vi "Example_chartsheet.vi"() -> ()   [LabVIEW 8.6]
uses:
  Controls/lxw_chart_marker_type.ctl
  Controls/lxw_chart_legend_position.ctl
  Controls/lxw_chart_axis_type.ctl
  Controls/lxw_chart_type.ctl
panel:
  out "function return 2":string
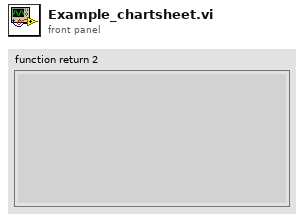
[diagram p1: front panel]
types:
  T1 = enum32{"invalid app kind", "Development System", "Run Time System", "Student Edition", "Embedded LabVIEW", "Evaluation", "Custom"}
  T2 = cluster{"color":u32, "none":u8, "@dummy control@":i8, "@dummy control@":i8, "@dummy control@":i8, "width":sgl, "dash_type":u8, "transparency":u8}
  T3 = cluster{"color":u32, "none":u8, "transparency":u8}
  T4 = typedef "lxw_chart_type.ctl" = u8
  T5 = typedef "lxw_chart_axis_type.ctl" = u8
  T6 = typedef "lxw_chart_legend_position.ctl" = u8
  T7 = typedef "lxw_chart_marker_type.ctl" = u8
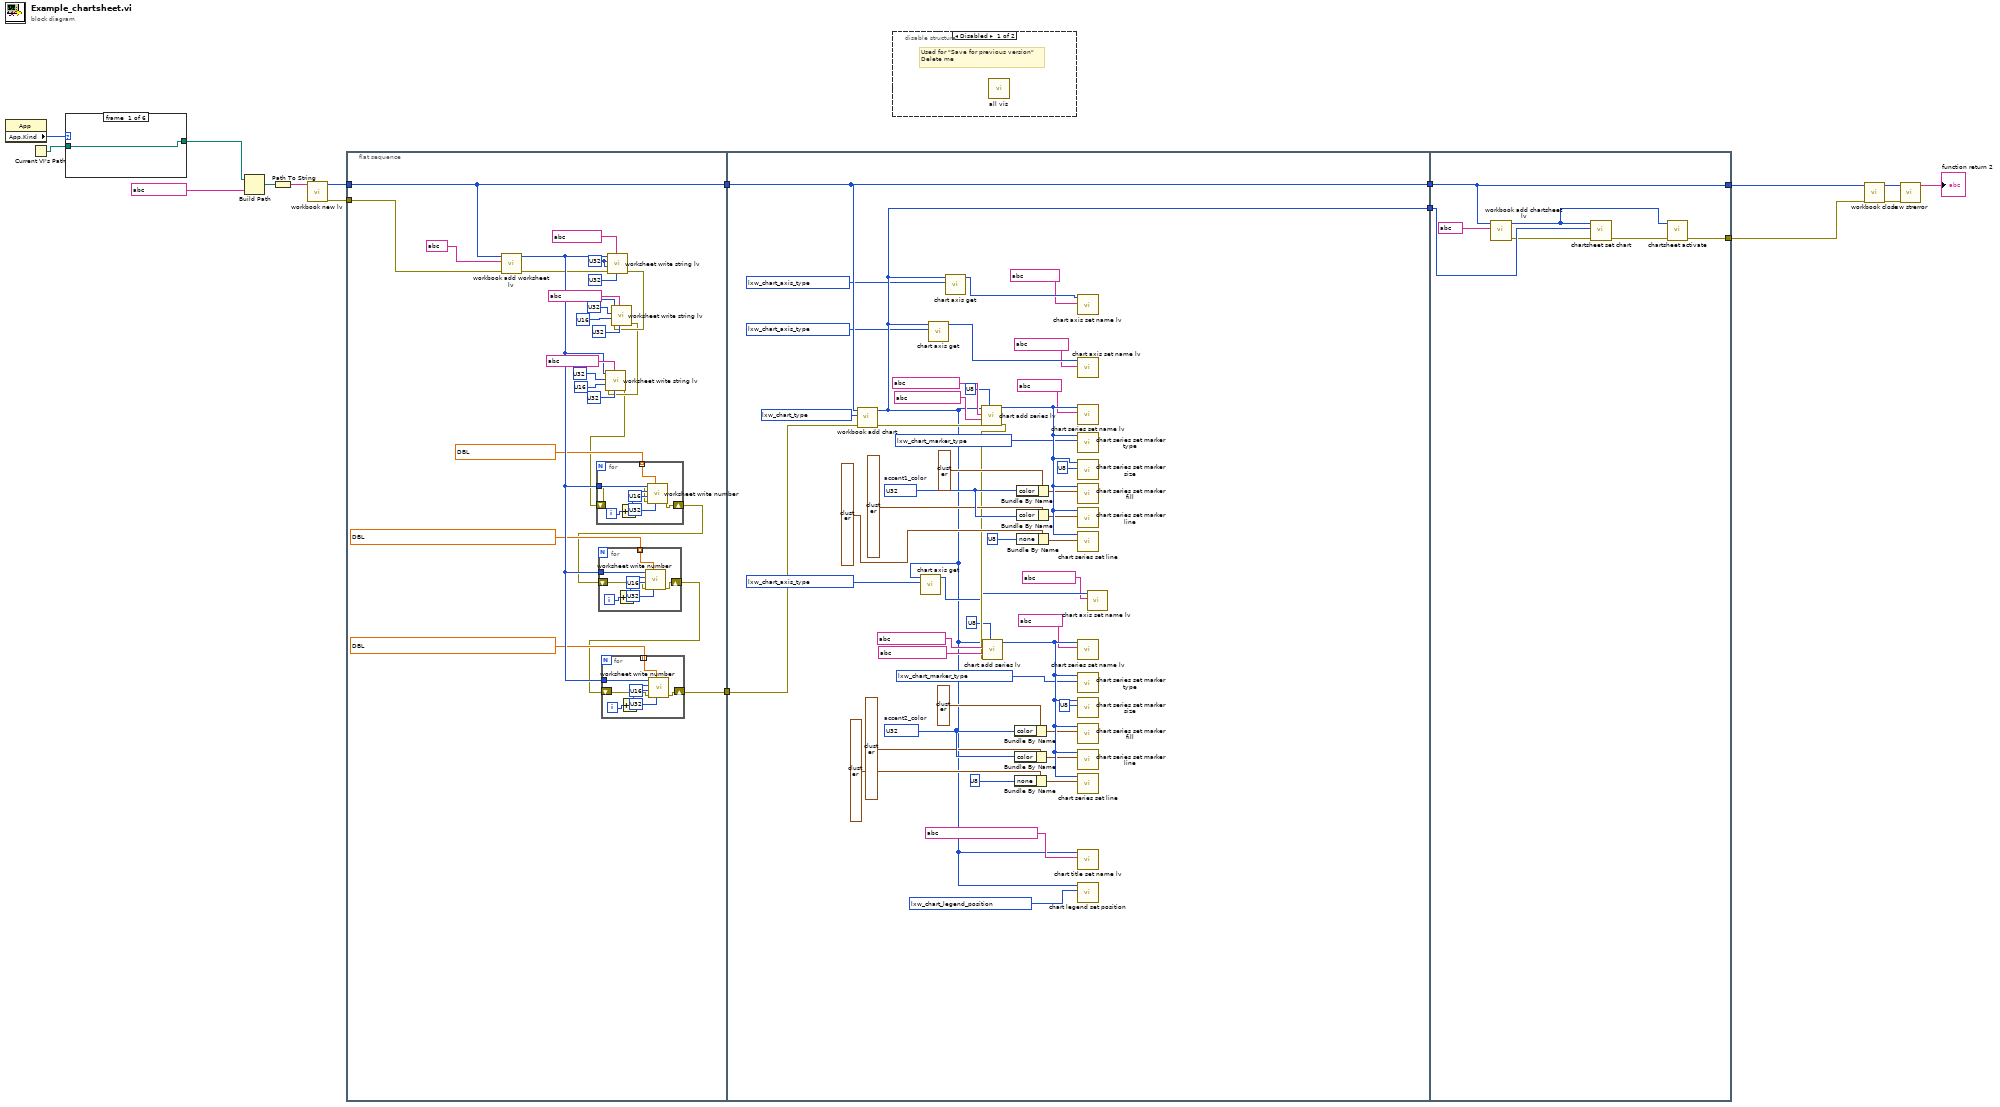
[diagram p0: block diagram]
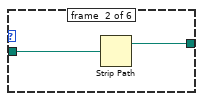
[diagram p2: hidden frame]
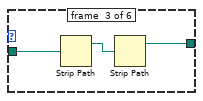
[diagram p3: hidden frame]
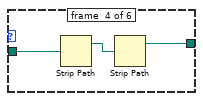
[diagram p4: hidden frame]
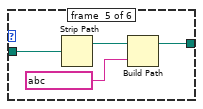
[diagram p5: hidden frame]
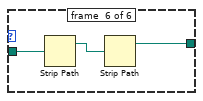
[diagram p6: hidden frame]
diagram:
  n1 = property class="App"() -> ("App.Kind"=w6:T1)  [unwired: 2 in, 2 out]
  n2 = Current VI's Path() -> (path=w5:path)
  n3 = case shown="\"Evaluation\"" w6 {
    tunnel: w5 -> [w18 w20 w23 w26 w30 w33]
    tunnel: [w18 w19 w21 w24 w28 w31] -> w3
    frame #0 {
    }
    frame #1 {
      n4 = Strip Path(path=w20) -> (stripped path=w19:path)  [unwired: 1 out]
    }
    frame #2 {
      n5 = Strip Path(path=w23) -> (stripped path=w22:path)  [unwired: 1 out]
      n6 = Strip Path(path=w22) -> (stripped path=w21:path)  [unwired: 1 out]
    }
    frame #3 {
      n7 = Strip Path(path=w26) -> (stripped path=w25:path)  [unwired: 1 out]
      n8 = Strip Path(path=w25) -> (stripped path=w24:path)  [unwired: 1 out]
    }
    frame #4 {
      n9 = Strip Path(path=w30) -> (stripped path=w29:path)  [unwired: 1 out]
      n10 = Build Path(base path=w29, name or relative path=string ?) -> (appended path=w28:path)
    }
    frame #5 {
      n11 = Strip Path(path=w33) -> (stripped path=w32:path)  [unwired: 1 out]
      n12 = Strip Path(path=w32) -> (stripped path=w31:path)  [unwired: 1 out]
    }
  }
  n13 = Build Path(base path=w3, name or relative path=string ? ("filename")) -> (appended path=w2:path)
  n14 = Path To String(path=w2) -> (string=w1:string)
  n15 = call "workbook new lv.vi"("filename"=w1) -> ("error out"=w14:errorcluster, "function return"=w17:u32)  [unwired: 9 in]
  n16 = flat-sequence {
    tunnel: w17 -> [w36]
    tunnel: w14 -> [w35]
    tunnel: [w37] -> w13
    tunnel: [w36] -> w12
    tunnel: w13 -> [w108]
    tunnel: w12 -> [w109]
    tunnel: [w109] -> w10
    tunnel: [w88] -> w9
    tunnel: [w135] -> w11
    tunnel: w10 -> [w133]
    tunnel: w9 -> [w134]
    tunnel: [w133] -> w8
    frame #0 {
      w57 = u32 ? ("row")
      n17 = call "workbook add worksheet lv.vi"("error in (no error)"=w35, "sheetname"=string ?, "workbook"=w36) -> ("error out"=w34:errorcluster, "function return"=w46:u32)  [unwired: 7 in]
      n18 = call "worksheet write string lv.vi"("format"=u32 ?, "string"=string ?, "error in (no error)"=w34, "col"=w57, "row"=w57, "worksheet"=w46) -> ("error out"=w42:errorcluster)  [unwired: 4 in, 1 out]
      n19 = call "worksheet write string lv.vi"("format"=u32 ?, "string"=string ?, "error in (no error)"=w42, "col"=u16 ?, "row"=u32 ?, "worksheet"=w46) -> ("error out"=w41:errorcluster)  [unwired: 4 in, 1 out]
      n20 = call "worksheet write string lv.vi"("format"=u32 ?, "string"=string ?, "error in (no error)"=w41, "col"=u16 ?, "row"=u32 ?, "worksheet"=w46) -> ("error out"=w40:errorcluster)  [unwired: 4 in, 1 out]
      n21 = for {
        tunnel: w46 -> [w82]
        tunnel: dbl[] ? -> [w81] mode=indexing
        shift-right: [w75] -> w39
        shift-left: w40 -> [w76]
        i -> [w80]
        n22 = Increment(x=w80) -> (x+1=w79:i32)
        n23 = call "worksheet write number.vi"("format"=u32 ?, "number"=w81, "error in (no error)"=w76, "col"=u16 ?, "row"=w79, "worksheet"=w82) -> ("error out"=w75:errorcluster)  [unwired: 4 in, 1 out]
      }
      n24 = for {
        tunnel: w46 -> [w74]
        tunnel: dbl[] ? -> [w73] mode=indexing
        shift-right: [w67] -> w38
        shift-left: w39 -> [w68]
        i -> [w72]
        n25 = Increment(x=w72) -> (x+1=w71:i32)
        n26 = call "worksheet write number.vi"("format"=u32 ?, "number"=w73, "error in (no error)"=w68, "col"=u16 ?, "row"=w71, "worksheet"=w74) -> ("error out"=w67:errorcluster)  [unwired: 4 in, 1 out]
      }
      n27 = for {
        tunnel: w46 -> [w66]
        tunnel: dbl[] ? -> [w65] mode=indexing
        shift-right: [w59] -> w37
        shift-left: w38 -> [w60]
        i -> [w64]
        n28 = Increment(x=w64) -> (x+1=w63:i32)
        n29 = call "worksheet write number.vi"("format"=u32 ?, "number"=w65, "error in (no error)"=w60, "col"=u16 ?, "row"=w63, "worksheet"=w66) -> ("error out"=w59:errorcluster)  [unwired: 4 in, 1 out]
      }
    }
    frame #1 {
      w83 = T4 ? items=["LXW_CHART_NONE", "LXW_CHART_AREA", "LXW_CHART_AREA_STACKED", "LXW_CHART_AREA_STACKED_PERCENT", "LXW_CHART_BAR", "LXW_CHART_BAR_STACKED", "LXW_CHART_BAR_STACKED_PERCENT", "LXW_CHART_COLUMN", "LXW_CHART_COLUMN_STACKED", "LXW_CHART_COLUMN_STACKED_PERCENT", "LXW_CHART_DOUGHNUT", "LXW_CHART_LINE", "LXW_CHART_LINE_STACKED", "LXW_CHART_LINE_STACKED_PERCENT", "LXW_CHART_PIE", "LXW_CHART_SCATTER", "LXW_CHART_SCATTER_STRAIGHT", "LXW_CHART_SCATTER_STRAIGHT_WITH_MARKERS", "LXW_CHART_SCATTER_SMOOTH", "LXW_CHART_SCATTER_SMOOTH_WITH_MARKERS", "LXW_CHART_RADAR", "LXW_CHART_RADAR_WITH_MARKERS", "LXW_CHART_RADAR_FILLED", "LXW_CHART_STOCK"] ("chart_type")
      w84 = T5 ? items=["LXW_CHART_AXIS_TYPE_X", "LXW_CHART_AXIS_TYPE_Y", "LXW_CHART_AXIS_TYPE_X2", "LXW_CHART_AXIS_TYPE_Y2"] ("axis_type")
      w85 = T5 ? items=["LXW_CHART_AXIS_TYPE_X", "LXW_CHART_AXIS_TYPE_Y", "LXW_CHART_AXIS_TYPE_X2", "LXW_CHART_AXIS_TYPE_Y2"] ("axis_type")
      w86 = T5 ? items=["LXW_CHART_AXIS_TYPE_X", "LXW_CHART_AXIS_TYPE_Y", "LXW_CHART_AXIS_TYPE_X2", "LXW_CHART_AXIS_TYPE_Y2"] ("axis_type")
      w90 = T6 ? items=["LXW_CHART_LEGEND_NONE", "LXW_CHART_LEGEND_RIGHT", "LXW_CHART_LEGEND_LEFT", "LXW_CHART_LEGEND_TOP", "LXW_CHART_LEGEND_BOTTOM", "LXW_CHART_LEGEND_TOP_RIGHT", "LXW_CHART_LEGEND_OVERLAY_RIGHT", "LXW_CHART_LEGEND_OVERLAY_LEFT"] ("position")
      w116 = T7 ? items=["LXW_CHART_MARKER_AUTOMATIC", "LXW_CHART_MARKER_NONE", "LXW_CHART_MARKER_SQUARE", "LXW_CHART_MARKER_DIAMOND", "LXW_CHART_MARKER_TRIANGLE", "LXW_CHART_MARKER_X", "LXW_CHART_MARKER_STAR", "LXW_CHART_MARKER_SHORT_DASH", "LXW_CHART_MARKER_LONG_DASH", "LXW_CHART_MARKER_CIRCLE", "LXW_CHART_MARKER_PLUS"] ("type")
      w115 = T7 ? items=["LXW_CHART_MARKER_AUTOMATIC", "LXW_CHART_MARKER_NONE", "LXW_CHART_MARKER_SQUARE", "LXW_CHART_MARKER_DIAMOND", "LXW_CHART_MARKER_TRIANGLE", "LXW_CHART_MARKER_X", "LXW_CHART_MARKER_STAR", "LXW_CHART_MARKER_SHORT_DASH", "LXW_CHART_MARKER_LONG_DASH", "LXW_CHART_MARKER_CIRCLE", "LXW_CHART_MARKER_PLUS"] ("type")
      w126 = u32 ?  # accent2_color
      w120 = u32 ?  # accent1_color
      n30 = call "workbook add chart.vi"("error in (no error)"=w108, "chart_type"=w83, "workbook"=w109) -> ("error out"=w107:errorcluster, "function return"=w88:u32)  [unwired: 7 in]
      n31 = call "chart axis get.vi"("axis_type"=w84, "chart"=w88) -> ("function return"=w93:u32)  [unwired: 8 in, 1 out]
      n32 = call "chart axis get.vi"("axis_type"=w85, "chart"=w88) -> ("function return"=w95:u32)  [unwired: 8 in, 1 out]
      n33 = call "chart axis get.vi"("axis_type"=w86, "chart"=w88) -> ("function return"=w97:u32)  [unwired: 8 in, 1 out]
      n34 = call "chart add series lv.vi"("y2_axis"=u8 ?, "error in (no error)"=w107, "values"=string ?, "categories"=string ?, "chart"=w88) -> ("error out"=w106:errorcluster, "function return"=w129:u32)  [unwired: 5 in]
      n35 = call "chart add series lv.vi"("y2_axis"=u8 ?, "error in (no error)"=w106, "values"=string ?, "categories"=string ?, "chart"=w88) -> ("function return"=w127:u32)  [unwired: 5 in, 1 out]
      n36 = Bundle By Name(cluster=T3 ? ("fill"), "color"=w126) -> (w100:T3)
      n37 = Bundle By Name(cluster=T2 ? ("line"), "color"=w126) -> (w98:T2)
      n38 = Bundle By Name(cluster=T2 ? ("line"), "none"=u8 ?) -> (w99:T2)
      n39 = Bundle By Name(cluster=T3 ? ("fill"), "color"=w120) -> (w104:T3)
      n40 = Bundle By Name(cluster=T2 ? ("line"), "color"=w120) -> (w103:T2)
      n41 = Bundle By Name(cluster=T2 ? ("line"), "none"=u8 ?) -> (w102:T2)
      n42 = call "chart axis set name lv.vi"("name"=string ?, "axis"=w97) -> ()  [unwired: 9 in, 1 out]
      n43 = call "chart axis set name lv.vi"("name"=string ?, "axis"=w95) -> ()  [unwired: 9 in, 1 out]
      n44 = call "chart series set name lv.vi"("name"=string ?, "series"=w129) -> ()  [unwired: 9 in, 1 out]
      n45 = call "chart series set marker type.vi"("type"=w115, "series"=w129) -> ()  [unwired: 9 in, 1 out]
      n46 = call "chart series set marker size.vi"("size"=u8 ?, "series"=w129) -> ()  [unwired: 9 in, 1 out]
      n47 = call "chart series set marker fill.vi"("fill"=w104, "series"=w129) -> ()  [unwired: 8 in, 2 out]
      n48 = call "chart series set marker line.vi"("line"=w103, "series"=w129) -> ()  [unwired: 8 in, 2 out]
      n49 = call "chart series set line.vi"("line"=w102, "series"=w129) -> ()  [unwired: 8 in, 2 out]
      n50 = call "chart series set name lv.vi"("name"=string ?, "series"=w127) -> ()  [unwired: 9 in, 1 out]
      n51 = call "chart series set marker type.vi"("type"=w116, "series"=w127) -> ()  [unwired: 9 in, 1 out]
      n52 = call "chart series set marker size.vi"("size"=u8 ?, "series"=w127) -> ()  [unwired: 9 in, 1 out]
      n53 = call "chart series set marker fill.vi"("fill"=w100, "series"=w127) -> ()  [unwired: 8 in, 2 out]
      n54 = call "chart series set marker line.vi"("line"=w98, "series"=w127) -> ()  [unwired: 8 in, 2 out]
      n55 = call "chart series set line.vi"("line"=w99, "series"=w127) -> ()  [unwired: 8 in, 2 out]
      n56 = call "chart title set name lv.vi"("name"=string ?, "chart"=w88) -> ()  [unwired: 9 in, 1 out]
      n57 = call "chart legend set position.vi"("position"=w90, "chart"=w88) -> ()  [unwired: 9 in, 1 out]
      n58 = call "chart axis set name lv.vi"("name"=string ?, "axis"=w93) -> ()  [unwired: 9 in, 1 out]
    }
    frame #2 {
      n59 = call "workbook add chartsheet lv.vi"("sheetname"=string ?, "workbook"=w133) -> ("error out"=w130:errorcluster, "function return"=w131:u32)  [unwired: 8 in]
      n60 = call "chartsheet set chart.vi"("error in (no error)"=w130, "chart"=w134, "chartsheet"=w131) -> ("error out"=w132:errorcluster)  [unwired: 7 in, 1 out]
      n61 = call "chartsheet activate.vi"("error in (no error)"=w132, "chartsheet"=w131) -> ("error out"=w135:errorcluster)  [unwired: 9 in]
    }
  }
  n62 = disable-structure shown="Disabled" {
    frame #0 {
      # "Used for \"Save for previous version\"\nDelete me"
      n63 = call "all vis.vi"() -> ()  [unwired: 12 in]
    }
    frame #1 {
    }
  }
  n64 = call "workbook close.vi"("error in (no error)"=w11, "workbook"=w8) -> ("error out"=w7:errorcluster, "function return"=w16:u32)  [unwired: 8 in]
  n65 = call "lxw strerror.vi"("error in (no error)"=w7, "error_num"=w16) -> ("function return"=→"function return 2":string)  [unwired: 8 in, 1 out]
